vi "Message Padding From First Pad Byte.vi"(1 "first pad byte":u8=6) -> (0 "string":string)   [LabVIEW 2020, in "NI_Keccak.lvlib"]
uses:
  <vilib>/security/Message Digest/Keccak/NI_Keccak.lvlib
  54930990-97ed-3fc8-5a55-36acfd26e33f.vi
  42b180f0-de70-3fd4-565d-d595c1a7ee3f.vi
  54930990-97ed-3fc8-5a55-36acfd26e33f.vi/100a7048-03ca-3fd8-5025-90e756c5df3f.vi
  54930990-97ed-3fc8-5a55-36acfd26e33f.vi/100a7048-03ca-3fd8-5025-90e756c5df3f.vi/3a7a0720-5fe7-3fc1-282a-afa83559cf3f.vi
  54930990-97ed-3fc8-5a55-36acfd26e33f.vi/100a7048-03ca-3fd8-5025-90e756c5df3f.vi/3a7a0720-5fe7-3fc1-282a-afa83559cf3f.vi/7d8c2d74-6d84-3fe6-2875-c0f7ea4fd63f.vi
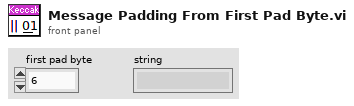
[diagram p1: front panel]
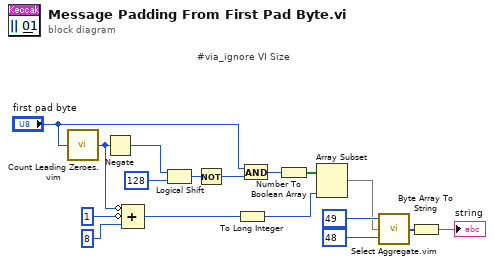
[diagram p0: block diagram]
diagram:
  # "#via_ignore VI Size"
  n1 = call "Count Leading Zeroes.vim"("x"="first pad byte") -> ("leading zeroes"=w5:i16)
  n2 = Negate(x=w5) -> (-x=w16:i16)
  n3 = Compound Arithmetic op=ADD(invert w5, invert i16 1 ("value"), i16 8 ("value")) -> (w2:i16)
  n4 = Logical Shift(y=w16, x=u8 128 ("first pad byte mask")) -> (x << y=w15:u8)
  n5 = Not(x=w15) -> (.not. x?=w14:u8)
  n6 = To Long Integer(number=w2) -> (32bit integer=w1:i32)
  n7 = And(x="first pad byte", y=w14) -> (x .and. y?=w13:u8)
  n8 = Number To Boolean Array(number=w13) -> (Boolean array=w7:bool[])
  n9 = Array Subset(array=w7, length=w1) -> (w6:bool[])  [unwired: 1 in]
  n10 = call "Select Aggregate.vim"("f"=u8 48 ("first pad byte mask"), "s"=w6, "t"=u8 49 ("first pad byte mask")) -> ("s?t:f"=w10:u8[])
  n11 = Byte Array To String(unsigned byte array=w10) -> (string=→"string":string)
